vi "empty_point_array.vi"() -> (0 "Array":cluster{"X":i32, "Y":i32}[](array[cluster]))   [LabVIEW 2017]
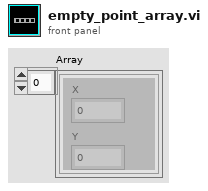
[diagram p1: front panel]
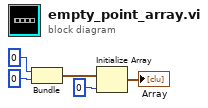
[diagram p0: block diagram]
diagram:
  n1 = Bundle(0, 0) -> (w5:cluster{i32, i32})  [unwired: 1 in]
  n2 = Initialize Array(w5, 0 ("dimension size")) -> (→"Array":cluster{i32, i32}[])
